vi "LiveFeed.vi"() -> ()   [LabVIEW 2024]
doc: "Drag this VI onto your front panel to load several icons that represent working code to display the image from a live video source (i.e. a webcam)."
uses:
  <userlib>/ImageProcessing/InitCamera_NTSC.vi
panel:
  in  "Stop":bool
  out "image":picture
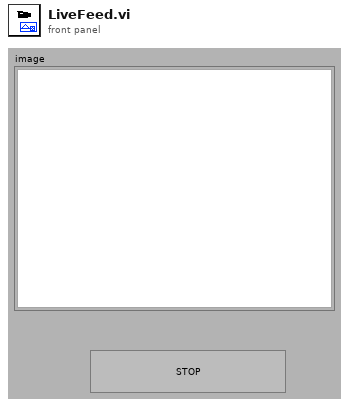
[diagram p1: front panel]
types:
  T1 = typedef "QT_Ref.ctl" = refnum<k1>
  T2 = typedef "QT_Image.ctl" = cluster{"Width":i32, "Height":i32, "Depth":i32, "data":u8[], "Compressed data":u8[], "Color table":u32[], "Duration":i32, "Options":i32, "Timestamp":i32, "ID":i32, "Reserved":i32, "Dialogs":u32}
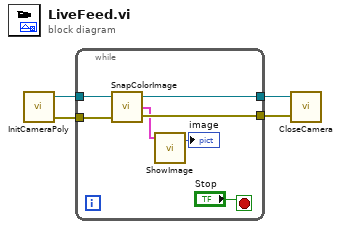
[diagram p0: block diagram]
diagram:
  n1 = call-poly <userlib>:"InitCameraPoly.vi"() -> ("error out"=w4:errorcluster, "QT Ref Out"=w3:T1)  [unwired: 2 in]
  n2 = while {
    tunnel: w4 -> [w11]
    tunnel: w3 -> [w10]
    tunnel: [w9] -> w2
    tunnel: [w8] -> w1
    stop <- "Stop" stop-if-true
    n3 = call <userlib>:"SnapColorImage.vi"("error in (no error)"=w11, "QT Ref In"=w10) -> ("error out"=w9:errorcluster, "Image Out"=w7:T2, "QT Ref Out"=w8:T1)  [unwired: 1 in]
    n4 = call <userlib>:"ShowImage.vi"("Image"=w7) -> ("image"=→"image":picture)  [unwired: 2 in, 1 out]
  }
  n5 = call <userlib>:"CloseCamera.vi"("error in (no error)"=w2, "QT Ref In"=w1) -> ()  [unwired: 1 in, 1 out]
